vi "combine array.vi"(6 "Previous Data":dbl[][](array[numeric]), 9 "X Values (solution)":dbl[][](array[numeric]), 10 "end element":i32, 11 "Times in":dbl[](array[numeric])) -> (2 "Index":i32, 3 "Combined Data":dbl[][](array[numeric]))   [LabVIEW 2025, in "Dynamic-System.lvclass"]
uses:
  Dynamic-System.lvclass
panel:
  in  "length":i32
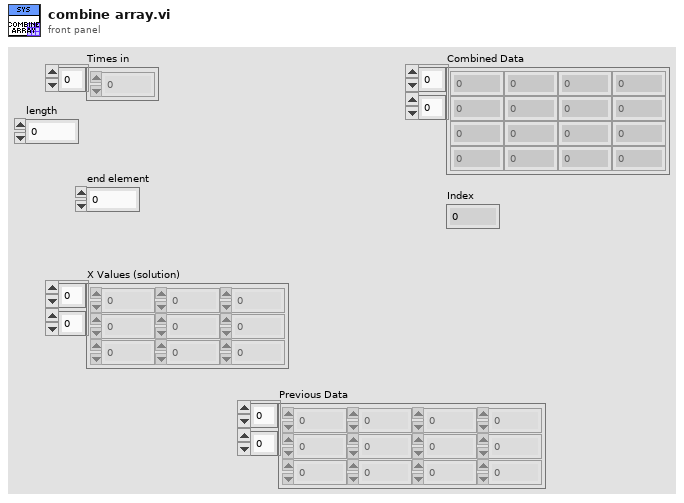
[diagram p1: front panel]
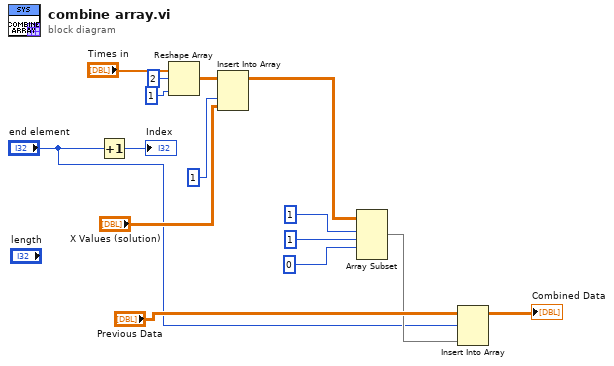
[diagram p0: block diagram]
diagram:
  n1 = Increment(x="end element") -> (x+1=→"Index":i32)
  n2 = Reshape Array("Times in", 2 ("dimension size"), 1 ("dimension size")) -> (w12:dbl[][])
  n3 = Insert Into Array(array=w12, index (col)=1 ("disabled index (col)"), new element="X Values (solution)") -> (w10:dbl[][])  [unwired: 1 in]
  n4 = Array Subset(array=w10, index (row)=1 ("index"), length (row)=1 ("length"), index (col)=0 ("index")) -> (w8:dbl[][])  [unwired: 1 in]
  n5 = Insert Into Array(array="Previous Data", index (row)="end element", new element=w8) -> (→"Combined Data":dbl[][])  [unwired: 1 in]
